vi "nQueen.vi"() -> ()   [LabVIEW 2014]
panel:
  out "All solutions in 3D array":bool[][][](array[boolean])
  in  "Display delay time(ms)":u32
  out "Solution counts":i32
  out "Solutions displayed by 2D array":bool[][](array[boolean])
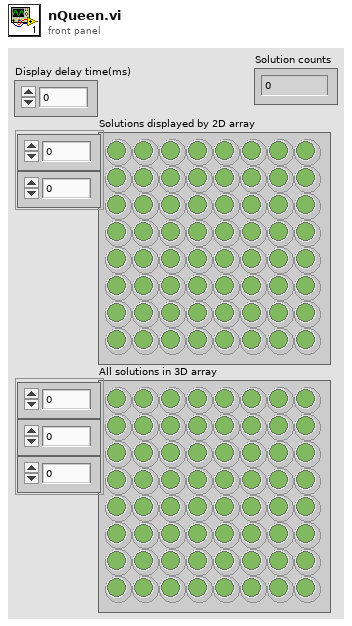
[diagram p1: front panel]
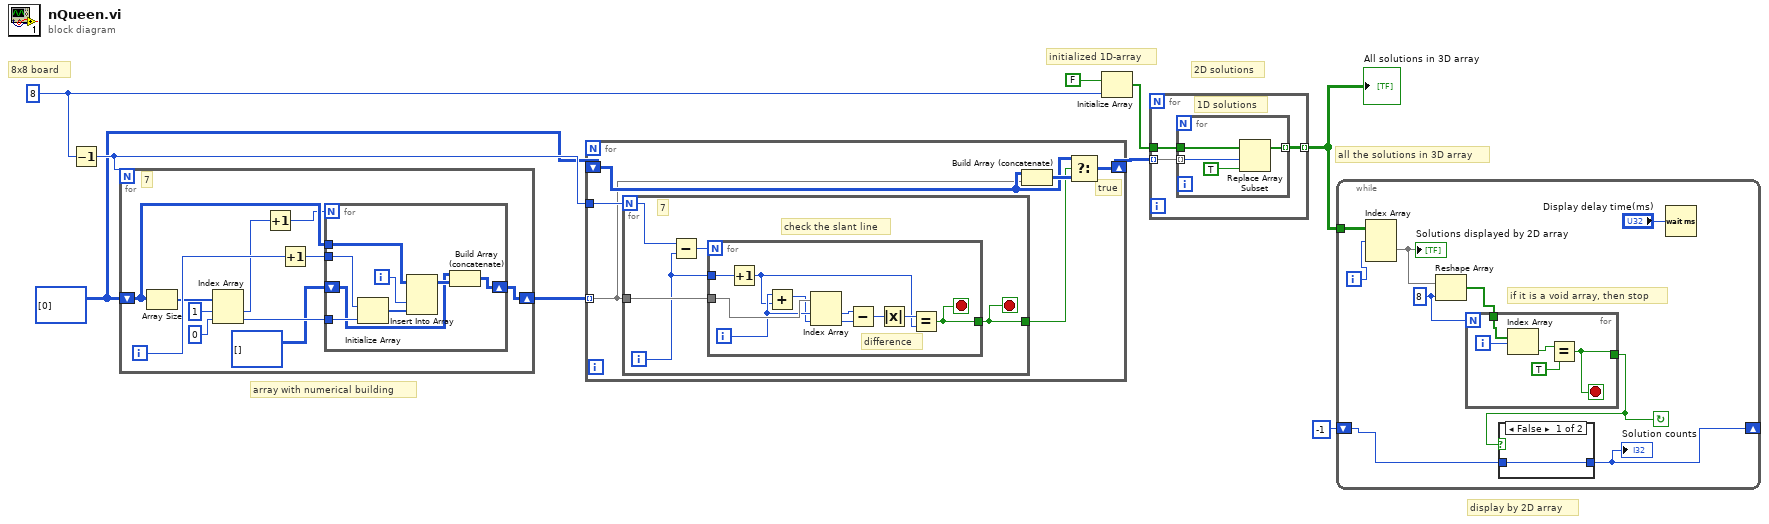
[diagram p0: block diagram]
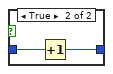
[diagram p2: hidden frame]
diagram:
  w3 = 8
  w2 = i32[][] [[0]] ("array")
  # "array with numerical building"
  # "display by 2D array"
  # "all the solutions in 3D array"
  # "2D solutions"
  # "initialized 1D-array"
  # "8x8 board"
  n1 = Decrement(x=w3) -> (x-1=w9:i32)
  n2 = for {
    N: w9 -> [_]
    shift-right: [w10] -> w8
    shift-left: w2 -> [w18]
    i -> [w20]
    # "7"
    n3 = Array Size(array=w18) -> (size(s)=w15:i32[])
    n4 = Index Array(array=w15, index #1=1 ("index"), index #2=0 ("index")) -> (element #1=w17:i32, element #2=w12:i32)
    n5 = Increment(x=w17) -> (x+1=w14:i32)
    n6 = Increment(x=w20) -> (x+1=w19:i32)
    n7 = for {
      N: w14 -> [_]
      tunnel: w19 -> [w27]
      tunnel: w18 -> [w25]
      tunnel: w12 -> [w28]
      shift-right: [w22] -> w10
      shift-left: i32[][] [] ("array") -> [w21]
      i -> [w26]
      n8 = Initialize Array(w27, w28) -> (w24:i32[])
      n9 = Insert Into Array(array=w25, index (col)=w26, new element=w24) -> (w23:i32[][])  [unwired: 1 in]
      n10 = Build Array (concatenate)(w21, w23) -> (w22:i32[][])
    }
  }
  n11 = for {
    tunnel: w8 -> [w29] mode=indexing
    tunnel: w9 -> [w31]
    shift-right: [w33] -> w5
    shift-left: w2 -> [w32]
    # "true"
    n12 = for {
      N: w31 -> [w38]
      tunnel: w29 -> [w39]
      tunnel: [w35] -> w30
      i -> [w36]
      stop <- w35 stop-if-true
      # "7"
      # "check the slant line"
      n13 = Subtract(x=w38, y=w36) -> (x-y=w37:i32)
      n14 = for {
        N: w37 -> [_]
        tunnel: w39 -> [w49]
        tunnel: w36 -> [w48]
        tunnel: [w40] -> w35
        i -> [w47]
        stop <- w40 stop-if-true
        # "difference"
        n15 = Increment(x=w48) -> (x+1=w41:i32)
        n16 = Add(x=w47, y=w41) -> (x+y=w46:i32)
        n17 = Index Array(array=w49, index #1=w47, index #2=w46) -> (element #1=w45:i32, element #2=w44:i32)
        n18 = Subtract(x=w45, y=w44) -> (x-y=w43:i32)
        n19 = Absolute Value(x=w43) -> (abs(x)=w42:i32)
        n20 = Equal?(x=w42, y=w41) -> (x = y?=w40:bool)
      }
    }
    n21 = Build Array (concatenate)(w32, w29) -> (w34:i32[][])
    n22 = Select(t=w32, s=w30, f=w34) -> (s? t:f=w33:i32[][])
  }
  n23 = Initialize Array(FALSE, w3) -> (w6:bool[])
  n24 = for {
    tunnel: w5 -> [w52] mode=indexing
    tunnel: [w51] -> w4 mode=indexing
    tunnel: w6 -> [w50]
    # "1D solutions"
    n25 = for {
      tunnel: w50 -> [w56]
      tunnel: w52 -> [w54] mode=indexing
      tunnel: [w53] -> w51 mode=indexing
      n26 = Replace Array Subset(array=w56, new element=TRUE, index=w54) -> (w53:bool[])
    }
  }
  "All solutions in 3D array" <- w4
  n27 = while {
    tunnel: w4 -> [w65]
    shift-right: [w58] -> _
    shift-left: -1 -> [w59]
    i -> [w64]
    stop <- w60 continue-if-true
    w62 = 8 ("dimension size")
    # "if it is a void array, then stop"
    n28 = Index Array(array=w65, index (dim 0)=w64) -> (element=w63:bool[][])  [unwired: 2 in]
    "Solutions displayed by 2D array" <- w63
    n29 = Reshape Array(w63, w62) -> (w61:bool[])
    n30 = for {
      N: w62 -> [_]
      tunnel: w61 -> [w72]
      tunnel: [w69] -> w60
      i -> [w73]
      stop <- w69 stop-if-true
      n31 = Index Array(array=w72, index=w73) -> (element=w71:bool)
      n32 = Equal?(x=w71, y=TRUE) -> (x = y?=w69:bool)
    }
    n33 = case shown="False" w60 {
      tunnel: w59 -> [w66 w68]
      tunnel: [w66 w67] -> w58
      frame False {
      }
      frame True {
        n34 = Increment(x=w68) -> (x+1=w67:i32)
      }
    }
    "Solution counts" <- w58
    n35 = Wait (ms)(milliseconds to wait="Display delay time(ms)") -> ()  [unwired: 1 out]
  }
